vi "FX3U&GA Code.vi"(0 "枚举":T1(ring), 1 "Read/Write":bool, 2 "PLC站号":string="05", 3 "PC号":string="FF", 4 "寄存器名":string="D", 5 "起始地址":string="1000", 7 "软元件个数":string="10", 9 "Write Data":string) -> (14 "Hex":string)   [LabVIEW 2014]
panel:
  # "可在PLC中设置"
  # "一般固定为FF"
  # "M/D"
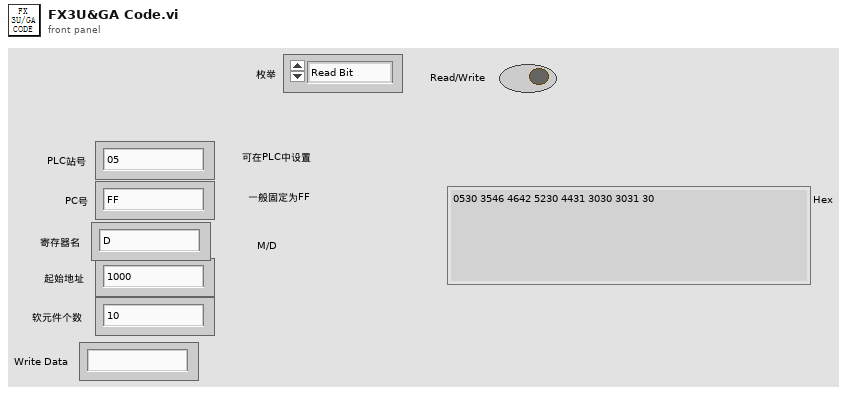
[diagram p1: front panel]
types:
  T1 = enum16{"Read Bit", "Read Word", "Write Bit", "Write Word"}
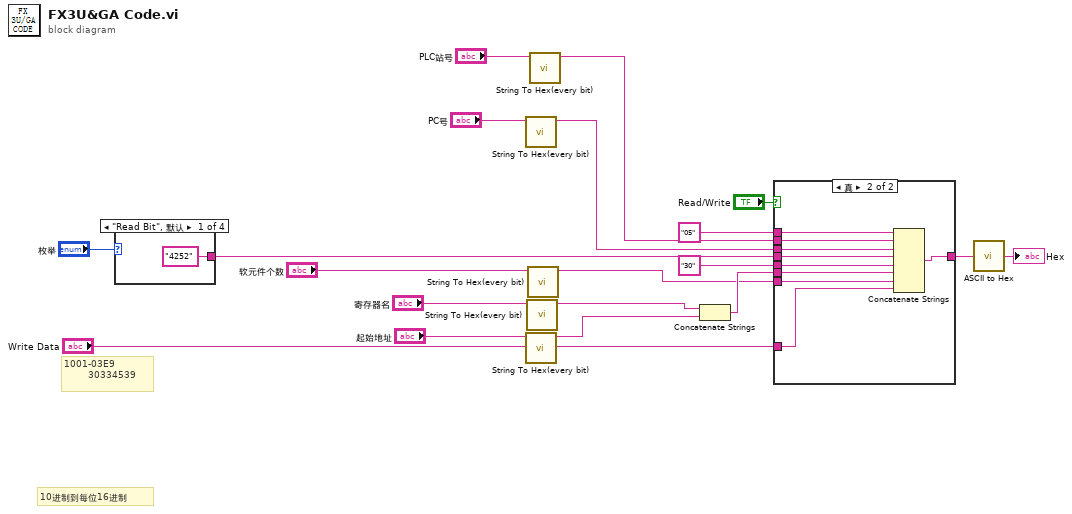
[diagram p0: block diagram]
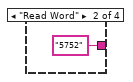
[diagram p2: hidden frame]
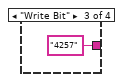
[diagram p3: hidden frame]
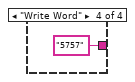
[diagram p4: hidden frame]
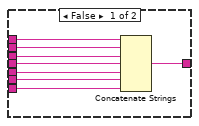
[diagram p5: hidden frame]
diagram:
  # "10进制到每位16进制"
  # "1001-03E9\n        30334539"
  n1 = case shown="\"Read Bit\", 默认" "枚举" {
    tunnel: ["4252" ("功能码") "5752" ("功能码") "4257" ("功能码") "5757" ("功能码")] -> w17
    frame "Read Bit", Default {
    }
    frame "Read Word" {
    }
    frame "Write Bit" {
    }
    frame "Write Word" {
    }
  }
  n2 = call "String To Hex(every bit).vi"("字符串"="PC号") -> ("十六进制整型字符串"=w7:string)  [unwired: 10 in]
  n3 = call "String To Hex(every bit).vi"("字符串"="起始地址") -> ("十六进制整型字符串"=w1:string)  [unwired: 10 in]
  n4 = call "String To Hex(every bit).vi"("字符串"="寄存器名") -> ("十六进制整型字符串"=w2:string)  [unwired: 10 in]
  n5 = call "String To Hex(every bit).vi"("字符串"="软元件个数") -> ("十六进制整型字符串"=w3:string)  [unwired: 10 in]
  n6 = call "String To Hex(every bit).vi"("字符串"="PLC站号") -> ("十六进制整型字符串"=w9:string)  [unwired: 10 in]
  n7 = Concatenate Strings(w2, w1) -> (w12:string)
  n8 = case shown="真" "Read/Write" {
    tunnel: [w31 w32] -> w19
    tunnel: "05" ("字符串") -> [w30 w40]
    tunnel: w9 -> [w29 w39]
    tunnel: w7 -> [w28 w38]
    tunnel: w17 -> [w27 w37]
    tunnel: "30" ("字符串") -> [w26 w36]
    tunnel: w12 -> [w25 w35]
    tunnel: w3 -> [w24 w34]
    tunnel: "Write Data" -> [_ w33]
    frame False {
      n9 = Concatenate Strings(w30, w29, w28, w27, w26, w25, w24) -> (w31:string)
    }
    frame True {
      n10 = Concatenate Strings(w40, w39, w38, w37, w36, w35, w34, w33) -> (w32:string)
    }
  }
  n11 = call "ASCII to Hex.vi"("ASCII"=w19) -> ("Hex"=→"Hex":string)
